vi "ReadControllerTemperature.vi"(11 "VISA resource name":refnum<visa-resource-name>="COM4") -> (0 "error out":errorcluster, 1 "Success?":bool, 3 "Temp":dbl format="%#_13g")   [LabVIEW 2022 SP3]
uses:
  <vilib>/Instr/_visa.llb/VISA Configure Serial Port (Instr).vi
panel:
  out "Return String":string
  out "BytesToRead":i32
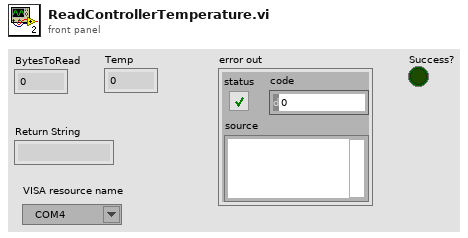
[diagram p1: front panel]
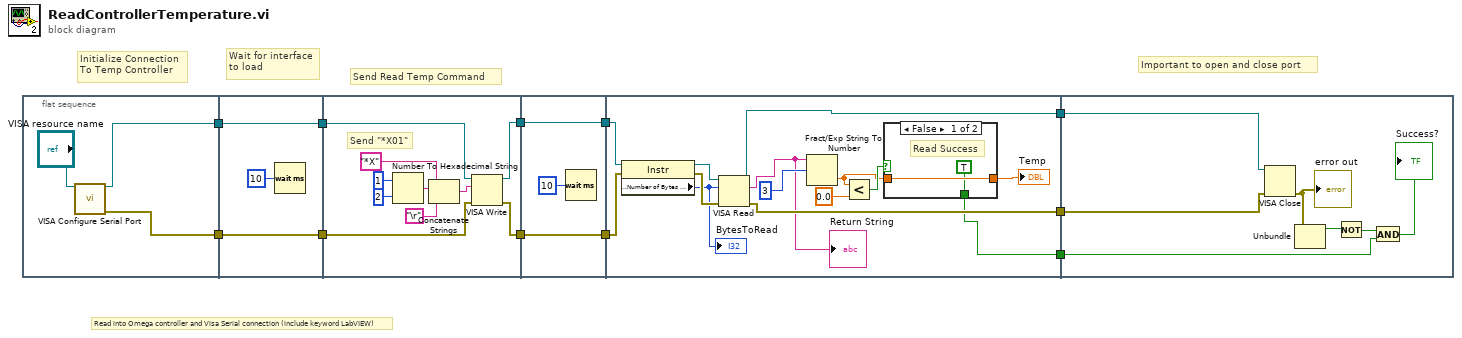
[diagram p0: block diagram]
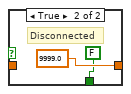
[diagram p2: hidden frame]
diagram:
  # "Important to open and close port"
  # "Read into Omega controller and Visa Serial connection (include keyword LabVIEW)"
  # "Initialize Connection\nTo Temp Controller"
  # "Wait for interface\nto load"
  # "Send Read Temp Command"
  n1 = flat-sequence {
    tunnel: [w14] -> w11
    tunnel: [w13] -> w10
    tunnel: w11 -> [w15]
    tunnel: w10 -> [w16]
    tunnel: [w16] -> w9
    tunnel: [w15] -> w8
    tunnel: w9 -> [w21]
    tunnel: w8 -> [w20]
    tunnel: [w19] -> w7
    tunnel: [w18] -> w6
    tunnel: w7 -> [w30]
    tunnel: w6 -> [w29]
    tunnel: [w30] -> w5
    tunnel: [w29] -> w4
    tunnel: w5 -> [w42]
    tunnel: w4 -> [w41]
    tunnel: [w39] -> w3
    tunnel: [w38] -> w2
    tunnel: [w31] -> w1
    tunnel: w3 -> [w55]
    tunnel: w2 -> [w54]
    tunnel: w1 -> [w50]
    frame #0 {
      n2 = call-poly "VISA Configure Serial Port"("VISA resource name"="VISA resource name") -> ("VISA resource name out"=w13:refnum<visa-resource-name>, "error out"=w14:errorcluster)  [unwired: 13 in]
    }
    frame #1 {
      n3 = Wait (ms)(milliseconds to wait=u32 10) -> ()  [unwired: 1 out]
    }
    frame #2 {
      # "Send \"*X01\""
      n4 = Number To Hexadecimal String(1:i16 2 ("width (-)"), 2:1 ("number")) -> (0:w25:string)
      n5 = Concatenate Strings("*X" ("string to write"), w25, "\r") -> (w22:string)
      n6 = VISA Write(VISA resource name=w21, write buffer=w22, error in (no error)=w20) -> (VISA resource name out=w19:refnum<visa-resource-name>, error out=w18:errorcluster)  [unwired: 1 out]
    }
    frame #3 {
      n7 = Wait (ms)(milliseconds to wait=u32 10) -> ()  [unwired: 1 out]
    }
    frame #4 {
      n8 = property class="Instr"(reference=w42, error in=w41) -> (reference out=w43:refnum<visa-resource-name>, error out=w44:errorcluster, "Serial Settings:Number of Bytes at Serial Port"=w37:u32)
      "BytesToRead" <- w37
      n9 = VISA Read(VISA resource name=w43, byte count=w37, error in (no error)=w44) -> (VISA resource name out=w39:refnum<visa-resource-name>, read buffer=w36:string, error out=w38:errorcluster)  [unwired: 1 out]
      "Return String" <- w36
      n10 = Fract/Exp String To Number(string=w36, offset=3) -> (number=w33:dbl)  [unwired: 2 in, 1 out]
      n11 = Less?(x=w33, y=0.0) -> (x < y?=w34:bool)
      n12 = case shown="False" w34 {
        tunnel: w33 -> [w46 _]
        tunnel: [w46 9999.0 ("y")] -> w32
        tunnel: [TRUE ("status") FALSE ("status")] -> w31
        frame False {
          # "Read Success"
        }
        frame True {
          # "Disconnected"
        }
      }
      "Temp" <- w32
    }
    frame #5 {
      n13 = VISA Close(VISA resource name=w55, error in (no error)=w54) -> (error out=w53:errorcluster)
      "error out" <- w53
      n14 = Unbundle(w53) -> ("status"=w52:bool)  [unwired: 2 out]
      n15 = Not(x=w52) -> (.not. x?=w51:bool)
      n16 = And(x=w51, y=w50) -> (x .and. y?=→"Success?":bool)
    }
  }
